vi "Validate Persistance.vi"(11 "Relation in":refnum<class "Relation.lvclass">) -> (0 "error out":errorcluster)   [LabVIEW 2020, in "Conditu2.lvlib" / "Columns.lvlib" / "Relation.lvclass"]
doc: "Ensures the mapping and nullable attribute is valid for the current value, returns an error otherwise.\n\nFor instance, if this is the many side of a OneToMany and the column isn't nullable but there's been no entity value set, then an error is returned. In order to not have a mapped entity linked, the column must be nullable."
uses:
  Relation.lvclass
  C:/dev/lv20CE/lv-conditum-tools/Conditum-Clone/Columns/Type/Type.lvclass
  Entity/Entity.lvclass
  Type/Type.lvclass/Type.ctl
  Relation.lvclass/Relation.ctl
  Type/Type.lvclass
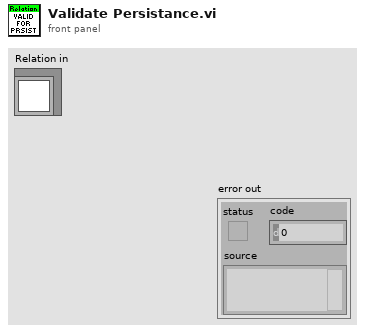
[diagram p1: front panel]
types:
  T1 = typedef "Conditu2.lvlib/Relation Mapping.ctl" = enum16{"OneToOne", "OneToMany", "ManyToOne", "ManyToMany"}
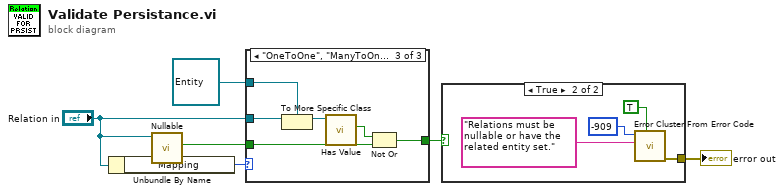
[diagram p0: block diagram]
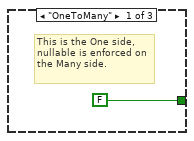
[diagram p2: hidden frame]
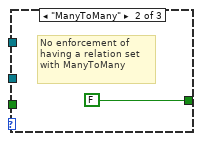
[diagram p3: hidden frame]
diagram:
  n1 = Unbundle By Name("Relation in") -> ("Mapping"=w6:T1)
  n2 = call "Nullable.vi"("Type in"="Relation in") -> ("Nullable"=w5:bool)  [unwired: 10 in]
  n3 = case shown="\"OneToOne\", \"ManyToOne\"" w6 {
    tunnel: w5 -> [_ _ w11]
    tunnel: "Relation in" -> [_ _ w14]
    tunnel: refnum<class "Entity.lvclass"> refnum ("Conditum:Columns:Entity.lvclass") -> [_ _ w13]
    tunnel: [FALSE FALSE w9] -> w2
    frame "OneToMany" {
      # "This is the One side, nullable is enforced on the Many side."
    }
    frame "ManyToMany" {
      # "No enforcement of having a relation set with ManyToMany"
    }
    frame "OneToOne", "ManyToOne" {
      n4 = To More Specific Class(target class=w13, reference=w14) -> (specific class reference=w12:refnum<class "Entity.lvclass">)  [unwired: 1 in, 1 out]
      n5 = call "Has Value.vi"("Entity in"=w12) -> ("Has Value"=w10:bool)  [unwired: 10 in]
      n6 = Not Or(1:w11, 2:w10) -> (0:w9:bool)
    }
  }
  n7 = case shown="True" w2 {
    tunnel: [_ w15] -> w1
    frame False {
    }
    frame True {
      n8 = call <vilib>:"Error Cluster From Error Code.vi"("show call chain? (False)"=TRUE, "error message (\"\")"="Relations must be nullable or have the related entity set." ("error message (\"\")"), "error code (0)"=-909) -> ("error out"=w15:errorcluster)  [unwired: 6 in]
    }
  }
  "error out" <- w1
